vi "Reliability System (FPGA).vi"() -> ()   [LabVIEW 2013]
uses:
  <vilib>/rvi/Emulation/niFpgaSctlEmulationGetInTimedLoop.vi
  <vilib>/rvi/Emulation/niFpgaEmulationReportErrorSimple.vi
  <vilib>/rvi/Emulation/niFpgaGetClockAttributes.vi
  <vilib>/rvi/eio/common/nirviEmuTemplateMethod_errors.vi
  <vilib>/rvi/Emulation/niFpgaCriticalErrorInLSC.vi
  <vilib>/rvi/interface/RandomDataEmulation/nirviRandomDataFPGAFIFO.vi
  <vilib>/rvi/interface/RandomDataEmulation/niFpgaRandomDataHandleErrors.vi
  <vilib>/eio/EIONode/EIONode.xnode
  <vilib>/rvi/FXPMathLib/FxpMul/XNode/nifxpmath_Multiplier.xnode
  <vilib>/rvi/FXPMathLib/FxpAdd/XNode/nifxpmath_Add.xnode
  <vilib>/rvi/DataTransferAndStorage/Container/XNode/niFpgaContainer.xnode
  <vilib>/rvi/interface/RandomDataEmulation/nirviRandomDataFpgaReadWriteTemplate.vi
  <vilib>/rvi/FXPMathLib/sim/FxpSim.dll
panel:
  out "Current Sweep":i16
  in  "Ht Cmd Offset":fxp<+/-,20,5> format="%#_17g"
  in  "Ht Cmd Slope":fxp<+/-,20,5>=1.0 format="%#_17g"
  out "Sweeps Running":bool
  out "Position Cmd Out":fxp<+/-,20,5>
  in  "Manual Cmd":bool
  in  "Start Sweep":bool
  in  "Sweep Count":i16
  in  "Total Samples":sgl format="%#_13g"
  in  "End Ht Cmd":sgl format="%#_13g"
  in  "Start Ht Cmd":sgl format="%#_13g"
  out "Height Read":fxp<+/-,24,5>
  in  "AO3 Spare":fxp<+/-,20,5>
  out "AI3 Spare":fxp<+/-,24,5>
  out "LS Voltage Read":fxp<+/-,24,5>
  out "PS Voltage Read":fxp<+/-,24,5>
  in  "PS Command":fxp<+/-,20,5>
  in  "Position Command":fxp<+/-,20,5>
  out "RMC/DI7":bool
  out "RMC/DI6":bool
  out "RMC/DI5":bool
  out "RMC/DI4":bool
  in  "RMC/DO3":bool
  in  "RMC/DO2":bool
  in  "RMC/DO1":bool
  in  "RMC/DO0":bool
  out "Height Raw":fxp<+/-,24,5>
  in  "100kHz Loop Control (us)":u32=10 caption="Count(uSec)"
  out "100kHz Loop Time (us)":u32
  out "10kHz Loop Time (us)":u32
  in  "10kHz Loop Control (us)":u32=100
  # "AO1\n(Emulated\nPosition)"
  # "AI2/10"
  # "AI1/9"
  # "AO0 (Position Command)"
  # "AI0/8"
  # "AO2"
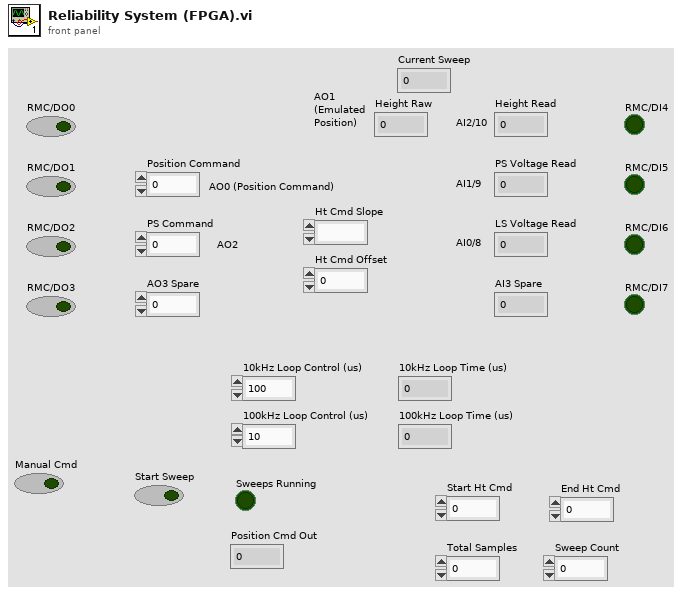
[diagram p1: front panel]
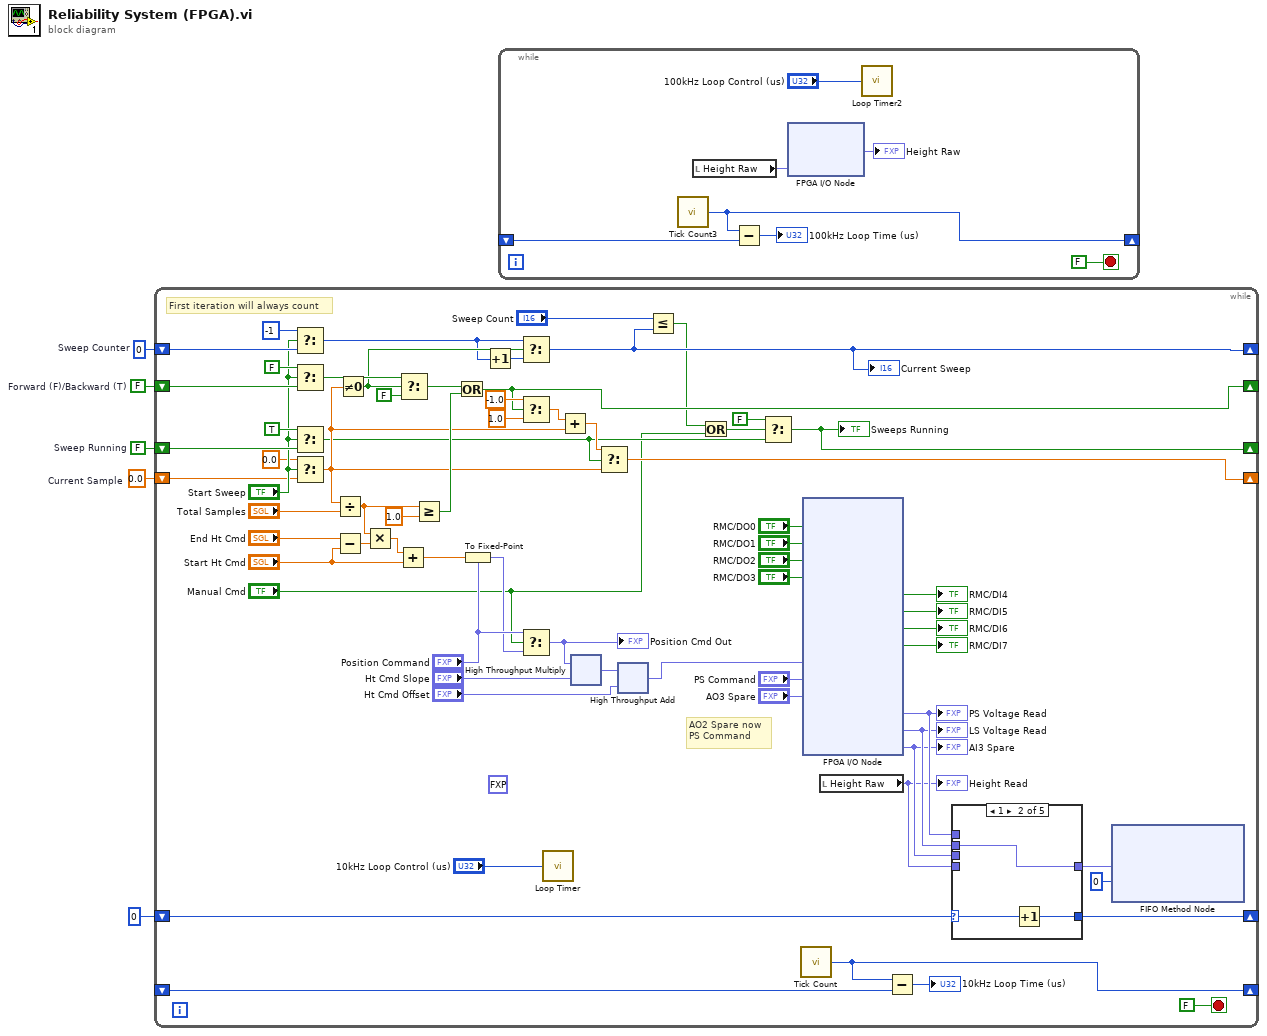
[diagram p0: block diagram]
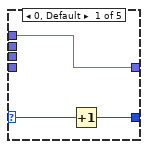
[diagram p2: hidden frame]
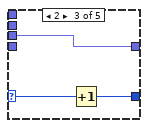
[diagram p3: hidden frame]
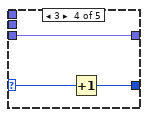
[diagram p4: hidden frame]
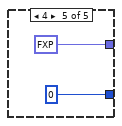
[diagram p5: hidden frame]
diagram:
  w1 = FALSE  # Sweep Running
  w2 = i16 0  # Sweep Counter
  w3 = FALSE  # Forward (F)/Backward (T)
  w4 = sgl 0.0  # Current Sample
  n1 = while {
    shift-right: [w71] -> _
    shift-left: _ -> [w70]
    shift-right: [w53] -> _
    shift-left: 0 ("Timeout") -> [w54]
    shift-right: [w37] -> _
    shift-left: w4 -> [w39]
    shift-right: [w30] -> _
    shift-left: w3 -> [w46]
    shift-right: [w20] -> _
    shift-left: w2 -> [w45]
    shift-right: [w17] -> _
    shift-left: w1 -> [w41]
    stop <- FALSE stop-if-true
    (unwired) fxp<+/-,20,5> 0.0 ("Ht Cmd Offset")
    # "First iteration will always count"
    # "AO2 Spare now\nPS Command"
    n2 = Select(t=i16 -1, s="Start Sweep", f=w45) -> (s? t:f=w23:i16)
    n3 = Select(t=FALSE, s="Start Sweep", f=w46) -> (s? t:f=w26:bool)
    n4 = Select(t=TRUE, s="Start Sweep", f=w41) -> (s? t:f=w18:bool)
    n5 = Select(t=sgl 0.0, s="Start Sweep", f=w39) -> (s? t:f=w28:sgl)
    n6 = Divide(x=w28, y="Total Samples") -> (x/y=w36:sgl)
    n7 = Subtract(x="End Ht Cmd", y="Start Ht Cmd") -> (x-y=w49:sgl)
    n8 = Not Equal To 0?(x=w28) -> (x != 0?=w24:bool)
    n9 = Multiply(x=w36, y=w49) -> (x*y=w50:sgl)
    n10 = Add(x=w50, y="Start Ht Cmd") -> (x+y=w14:sgl)
    n11 = Select(t=w26, s=w24, f=FALSE) -> (s? t:f=w25:bool)
    n12 = Greater Or Equal?(x=w36, y=sgl 1.0) -> (x >= y?=w34:bool)
    n13 = Or(x=w25, y=w34) -> (x .or. y?=w30:bool)
    n14 = To Fixed-Point(fixed-point type="Position Command", number=w14) -> (fixed-point=w12:fxp<+/-,20,5>)
    n15 = Increment(x=w23) -> (x+1=w22:i16)
    n16 = Select(t=w23, s=w24, f=w22) -> (s? t:f=w20:i16)
    "Current Sweep" <- w20
    n17 = Select(t=sgl -1.0, s=w30, f=sgl 1.0) -> (s? t:f=w29:sgl)
    n18 = Select(t="Position Command", s="Manual Cmd", f=w12) -> (s? t:f=w7:fxp<+/-,20,5>)
    "Position Cmd Out" <- w7
    n19 = call "Loop Timer"("Count(uSec)"="10kHz Loop Control (us)") -> ()  [unwired: 1 out]
    n20 = Add(x=w29, y=w28) -> (x+y=w33:sgl)
    n21 = xnode "High Throughput Multiply"("x"=w7, "y"="Ht Cmd Slope") -> ("x*y"=w9:fxp<+/-,40,10>)
    n22 = Select(t=w33, s=w18, f=w28) -> (s? t:f=w37:sgl)
    n23 = xnode "High Throughput Add"("x"=w9, "y"="Ht Cmd Offset") -> ("x+y"=w6:fxp<+/-,41,11>)
    n24 = Less Or Equal?(x="Sweep Count", y=w20) -> (x <= y?=w16:bool)
    n25 = Or(x=w16, y="Manual Cmd") -> (x .or. y?=w15:bool)
    n26 = Select(t=FALSE, s=w15, f=w18) -> (s? t:f=w17:bool)
    "Sweeps Running" <- w17
    n27 = call "Tick Count"() -> ("Tick Count(uSec)"=w71:u32)
    n28 = xnode "FPGA I/O Node"("RMC/DIO0"="RMC/DO0", "RMC/DIO1"="RMC/DO1", "RMC/DIO2"="RMC/DO2", "RMC/DIO3"="RMC/DO3", "AO0"=w6, "AO2"="PS Command", "AO3"="AO3 Spare") -> ("RMC/DIO4"=→"RMC/DI4":bool, "RMC/DIO5"=→"RMC/DI5":bool, "RMC/DIO6"=→"RMC/DI6":bool, "RMC/DIO7"=→"RMC/DI7":bool, "AI1"=w58:fxp<+/-,24,5>, "AI0"=w57:fxp<+/-,24,5>, "AI3"=w56:fxp<+/-,24,5>)  [unwired: 14 in, 14 out]
    "PS Voltage Read" <- w58
    "LS Voltage Read" <- w57
    "AI3 Spare" <- w56
    n29 = local read "Height Raw"() -> (w55:fxp<+/-,24,5>)
    "Height Read" <- w55
    n30 = Subtract(x=w71, y=w70) -> (x-y=→"10kHz Loop Time (us)":u32)
    n31 = case shown="1" w54 {
      selector: w54 -> [w77 w80 w83 w86 _]
      tunnel: w58 -> [w75 _ _ _ _]
      tunnel: w57 -> [_ w78 _ _ _]
      tunnel: w56 -> [_ _ w81 _ _]
      tunnel: w55 -> [_ _ _ w84 _]
      tunnel: [w76 w79 w82 w85 0 ("Timeout")] -> w53
      tunnel: [w75 w78 w81 w84 fxp<+/-,24,5> -15.0 ("Height Raw")] -> w52
      frame 0, Default {
        n32 = Increment(x=w77) -> (x+1=w76:i32)
      }
      frame 1 {
        n33 = Increment(x=w80) -> (x+1=w79:i32)
      }
      frame 2 {
        n34 = Increment(x=w83) -> (x+1=w82:i32)
      }
      frame 3 {
        n35 = Increment(x=w86) -> (x+1=w85:i32)
      }
      frame 4 {
      }
    }
    n36 = xnode ("FIFO Method Node")("Element"=w52, "Timeout"=0) -> ()  [unwired: 1 in, 2 out]
  }
  n37 = while {
    shift-right: [w93] -> _
    shift-left: _ -> [w94]
    stop <- FALSE stop-if-true
    n38 = call "Tick Count3"() -> ("Tick Count(uSec)"=w93:u32)
    n39 = local read "Height Raw"() -> (w89:fxp<+/-,24,5>)
    n40 = Subtract(x=w93, y=w94) -> (x-y=→"100kHz Loop Time (us)":u32)
    n41 = xnode "FPGA I/O Node"("AO1"=w89) -> ("AI2"=→"Height Raw":fxp<+/-,24,5>)  [unwired: 2 in, 2 out]
    n42 = call "Loop Timer2"("Count(uSec)"="100kHz Loop Control (us)") -> ()  [unwired: 1 out]
  }
